vi "Write Nibble.vi"(8 "error in (no error)":errorcluster, 9 "Value":u8 format="%.0x", 10 "Session in":refnum<class "Session.lvclass">, 11 "PCF8574 I2C LCD in":refnum<class "PCF8574 I2C LCD.lvclass">) -> (0 "error out":errorcluster, 2 "Session out":refnum<class "Session.lvclass">, 3 "PCF8574 I2C LCD out":refnum<class "PCF8574 I2C LCD.lvclass">)   [LabVIEW 2020, in "CTI-Peripheral.lvlib" / "PCF8574 I2C LCD.lvclass"]
uses:
  PCF8574 I2C LCD.lvclass
  CTI/Session/Session.lvclass
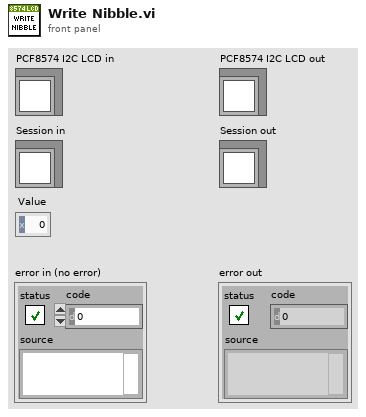
[diagram p1: front panel]
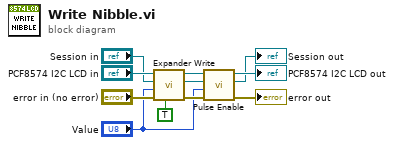
[diagram p0: block diagram]
diagram:
  n1 = call "Expander Write.vi"("NoStop (F)"=TRUE, "error in (no error)"="error in (no error)", "Value"="Value", "Session in"="Session in", "PCF8574 I2C LCD in"="PCF8574 I2C LCD in") -> ("error out"=w10:errorcluster, "Session out"=w4:refnum<class "Session.lvclass">, "PCF8574 I2C LCD out"=w6:refnum<class "PCF8574 I2C LCD.lvclass">)  [unwired: 4 in]
  n2 = call "Pulse Enable.vi"("error in (no error)"=w10, "Value"="Value", "Session in"=w4, "PCF8574 I2C LCD in"=w6) -> ("error out"=→"error out":errorcluster, "Session out"=→"Session out":refnum<class "Session.lvclass">, "PCF8574 I2C LCD out"=→"PCF8574 I2C LCD out":refnum<class "PCF8574 I2C LCD.lvclass">)  [unwired: 5 in]
